vi "Pcre2GetCodePointer8.vi"(8 "error in":errorcluster, 11 "pMatchData":u64 format="%.0x") -> (0 "error out":errorcluster, 2 "pCode":u64 format="%.0x", 3 "pMatchData":u64 format="%.0x")   [LabVIEW 2021, in "libpcre2-8.lvlib"]
uses:
  libpcre2-8.lvlib
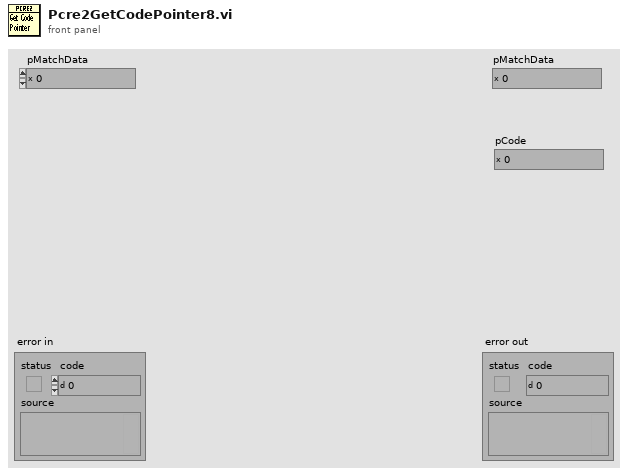
[diagram p1: front panel]
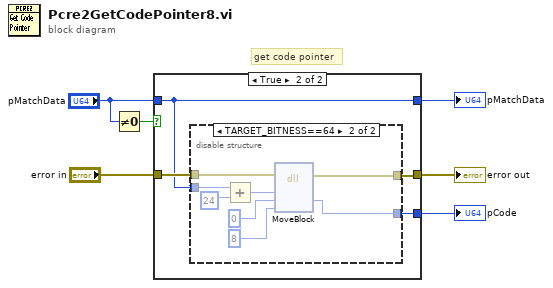
[diagram p0: block diagram]
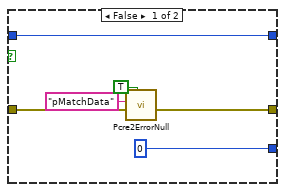
[diagram p2: hidden frame]
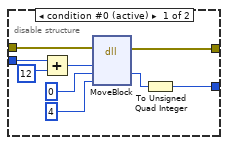
[diagram p3: hidden frame]
diagram:
  # "get code pointer"
  n1 = Not Equal To 0?(x="pMatchData") -> (x != 0?=w2:bool)
  n2 = case shown="True" w2 {
    tunnel: "error in" -> [w9 w16]
    tunnel: [w12 w13] -> w5
    tunnel: [w10 w15] -> w4
    tunnel: [u64 0 ("pointerDest") w14] -> w1
    tunnel: "pMatchData" -> [w12 w13]
    frame False {
      n3 = call "Pcre2ErrorNull.vi"("IsPointer? (F)"=TRUE, "error in"=w9, "What"="pMatchData") -> ("error out"=w10:errorcluster)  [unwired: 8 in]
    }
    frame True {
      n4 = disable-structure shown="TARGET_BITNESS==64" {
        disable-tunnel: w16 -> [w22 w30]
        disable-tunnel: [w21 w29] -> w15
        disable-tunnel: [w17 w28] -> w14
        disable-tunnel: w13 -> [w18 w26]
        frame condition #0 (active) {
          n5 = Add(x=w18, y=u64 12) -> (x+y=w25:u64)
          n6 = dll-call lib="LabVIEW" fn="MoveBlock"(error in=w22, "pointerSrc"=w25, "pointerDest"=u32 0 ("size"), "size"=u64 4) -> (error out=w21:errorcluster, "pointerDest"=w20:u32)  [unwired: 5 in, 1 out]
          n7 = To Unsigned Quad Integer(1:w20) -> (0:w17:u64)
        }
        frame condition #1 {
          n8 = Add(x=w26, y=u64 24) -> (x+y=w33:u64)
          n9 = dll-call lib="LabVIEW" fn="MoveBlock"(error in=w30, "pointerSrc"=w33, "pointerDest"=u64 0 ("size"), "size"=u64 8) -> (error out=w29:errorcluster, "pointerDest"=w28:u64)  [unwired: 5 in, 1 out]
        }
      }
    }
  }
  "pMatchData" <- w5
  "error out" <- w4
  "pCode" <- w1
